vi "Drive Loop Command.vi"   [LabVIEW 2015]
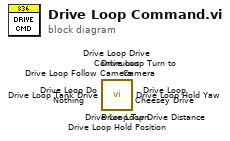
[diagram p0: block diagram]
diagram:
  n1 = call <userlib>:"Drive Loop Turn.vi"() -> ()  [unwired: 12 in]
  n2 = call <userlib>:"Drive Loop Turn to Camera.vi"() -> ()  [unwired: 12 in]
  n3 = call <userlib>:"Drive Loop Tank Drive.vi"() -> ()  [unwired: 12 in]
  n4 = call <userlib>:"Drive Loop Hold Yaw.vi"() -> ()  [unwired: 12 in]
  n5 = call <userlib>:"Drive Loop Hold Position.vi"() -> ()  [unwired: 12 in]
  n6 = call <userlib>:"Drive Loop Follow Camera.vi"() -> ()  [unwired: 12 in]
  n7 = call <userlib>:"Drive Loop Drive Distance.vi"() -> ()  [unwired: 12 in]
  n8 = call <userlib>:"Drive Loop Drive Continuous.vi"() -> ()  [unwired: 12 in]
  n9 = call <userlib>:"Drive Loop Do Nothing.vi"() -> ()  [unwired: 12 in]
  n10 = call <userlib>:"Drive Loop Cheesey Drive.vi"() -> ()  [unwired: 12 in]
